vi "Get All Data Names - When File Is Empty - Returns Empty Array.vi"() -> ()   [LabVIEW 2017]
uses:
  Json Data Reader/Json Data Reader.lvclass
  Assertion/Assertion.lvlib
panel:
  out "error out":errorcluster
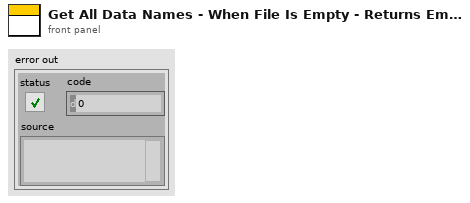
[diagram p1: front panel]
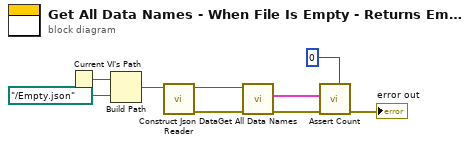
[diagram p0: block diagram]
diagram:
  n1 = Current VI's Path() -> (path=w3:path)
  n2 = Build Path(base path=w3, name or relative path=path "../Empty.json") -> (appended path=w1:path)
  n3 = call "Construct Json Data Reader.vi"("Json File"=w1) -> ("error out"=w8:errorcluster, "Json Data Reader"=w9:refnum<class "Json Data Reader.lvclass">)  [unwired: 9 in]
  n4 = call "Get All Data Names.vi"("error in (no error)"=w8, "Json Data Reader in"=w9) -> ("error out"=w7:errorcluster, "Test Data"=w6:cluster{"name":string, "<JSON>data":string}[])  [unwired: 7 in, 1 out]
  n5 = call "Assert Count.vi"("Expected"=0, "error in (no error)"=w7, "Haystack"=w6) -> ("error out"=→"error out":errorcluster)  [unwired: 8 in]
